vi "Balance_Sweep_Client.vi"(3 "Mode":bool, 4 "Measurement Time (ms)":i32, 5 "Stop Angle":dbl) -> (1 "Data Out":string)   [LabVIEW 2022 SP3]
uses:
  OGI_Server/ATE_Balance_Data.ctl
  Globals/Trav_pos_global.vi
  <vilib>/Platform/TimedLoop/XDataNode/XDataNode.xnode
  <vilib>/Platform/TimedLoop/XDataNode/timing_clust.ctl
  <vilib>/Platform/TimedLoop/XDataNode/wakeup.ctl
  <vilib>/Platform/TimedLoop/XDataNode/nitl_modes.ctl
  OGI_Server/ATE_Fan_Data.ctl
  <userlib>/LV-Link3/PolySubVIs/DtCreateAoutChan.vi
  <userlib>/LV-Link3/PolySubVIs/DtOLWriteSingle.vi
panel:
  out "Measurement Time":i32
  out "Initial":i64
  out "Target Angle":dbl
  out "Sampling Frequency":dbl
  out "DT Error":errorcluster
  out "Task out":i32
  out "Fan Data Ref":refnum<k21>
  out "Live Angle":dbl
  out "Balance Data Ref":refnum<k21>
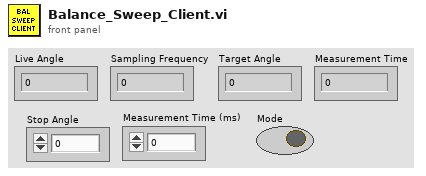
[diagram p1: front panel]
types:
  T1 = enum32{"Bad", "Idle", "Run top level", "Running"}
  T2 = typedef "XDNodeRunTimeDep.lvlib/timing_clust.ctl" = cluster{"Expected End [f-1]":u64, "Actual End [f-1]":u64, "Finished Late? [f-1]":bool, "Expected End [i-1]":u64, "Actual End [i-1]":u64, "Finished Late? [i-1]":bool, "Expected Start [i]":u64, "Actual Start [i]":u64, "Expected Start [f]":u64, "Actual Start [f]":u64, "Source Name":string, "Structure Name":string, "Period":i64, "Deadline":i64, "Offset":i64, "Start":i64, "Priority":i32, "Timeout":i32, "Mode":T3, "Wakeup Reason":T4, "Error":errorcluster, "Source Type":string, "Secondary Source Type":string, "Global End Time":u64, "Global Start Time":u64, "Frame Duration":u64, "Iteration Duration":u64, "Assigned CPU":i32, "I/O Scan Engine Mode":u32}
  T3 = typedef "XDNodeRunTimeDep.lvlib/nitl_modes.ctl" = enum32{"No Change", "Process missed periods, maintain original phase", "Discard missed periods, maintain original phase", "Process missed periods, ignore original phase", "Discard missed periods, ignore original phase"}
  T4 = typedef "XDNodeRunTimeDep.lvlib/wakeup.ctl" = enum32{"Normal", "Aborted", "Asynchronous wakeup", "Timing source error", "Timed loop error", "Timeout"}
  T5 = enum16{"big-endian, network order", "native, host order", "little-endian"}
  T6 = typedef "ATE_Fan_Data.ctl" = cluster{"Fan Speed (RPM)":dbl, "Wind Speed (m/s)":dbl, "SMAD Data":string}
  T7 = typedef "ATE_Balance_Data.ctl" = cluster{"%Lift":dbl, "Lift":dbl, "%Pitch":dbl, "Pitch":dbl, "%Drag":dbl, "Drag":dbl, "%Side":dbl, "Side":dbl, "%Yaw":dbl, "Yaw":dbl, "%Roll":dbl, "Roll":dbl}
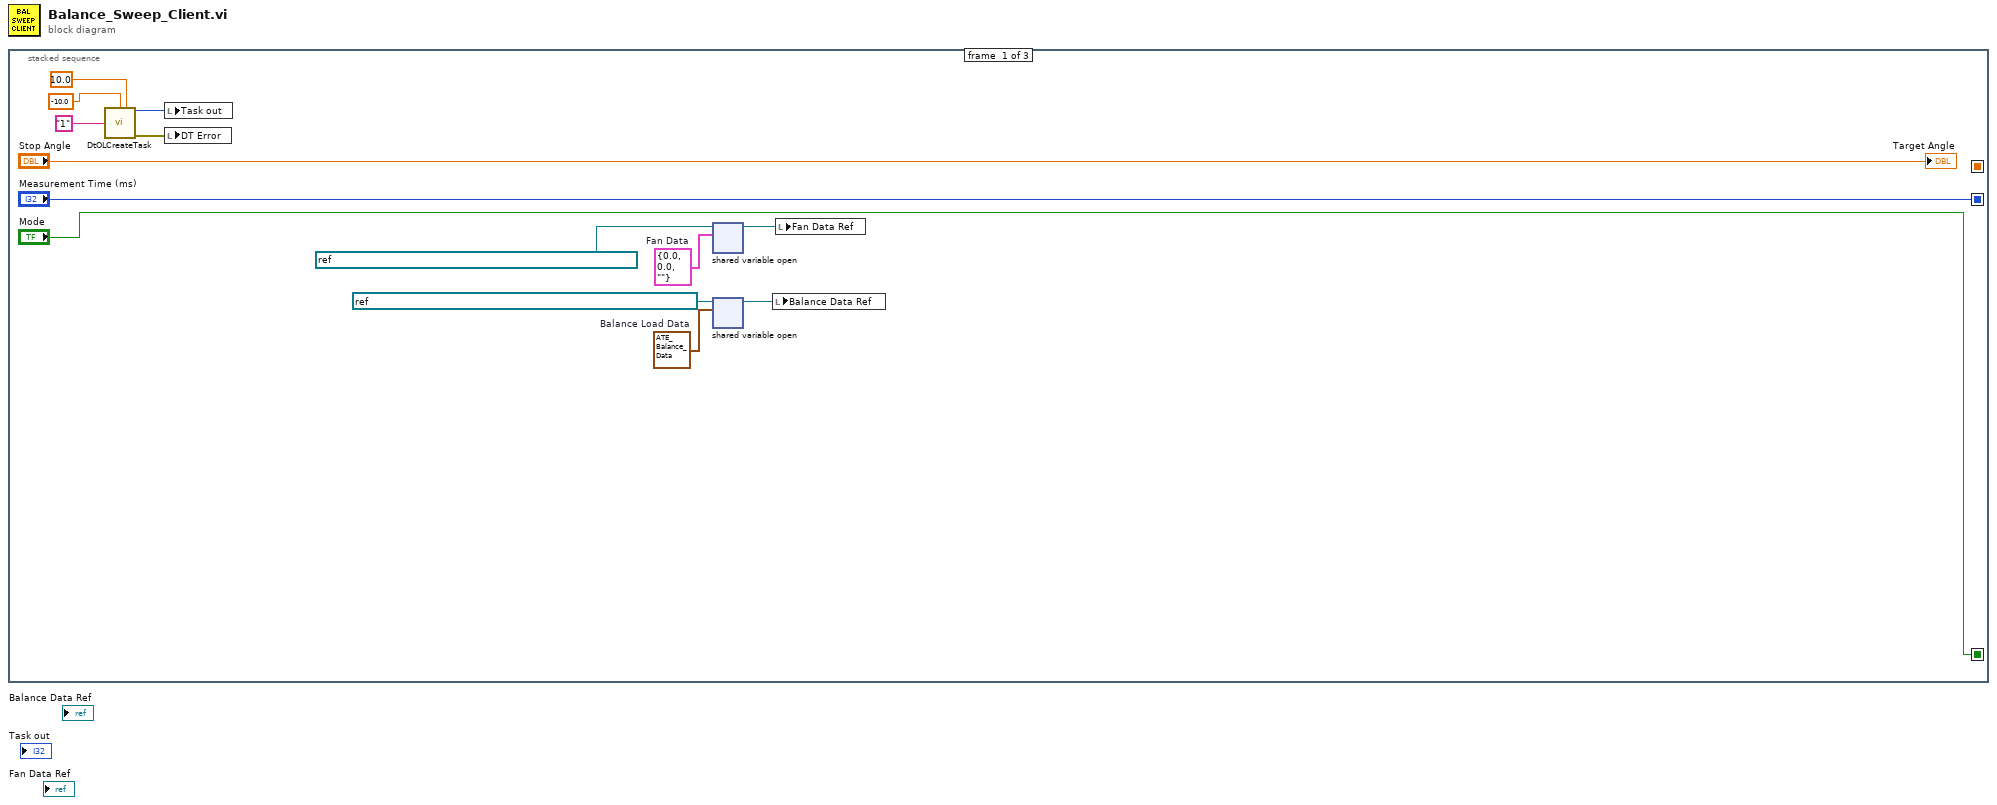
[diagram p0: block diagram]
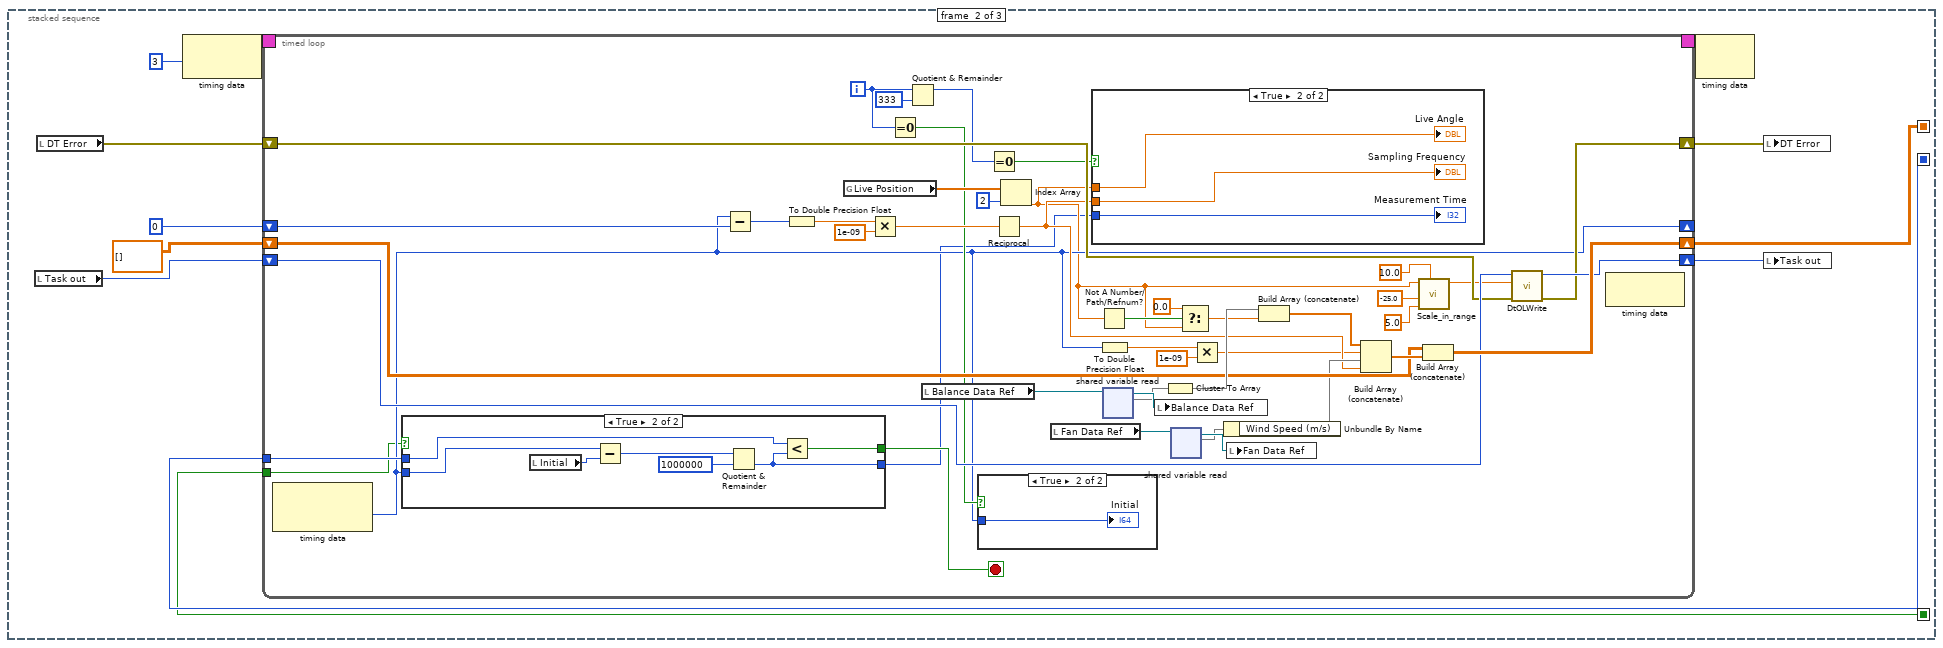
[diagram p2: hidden frame]
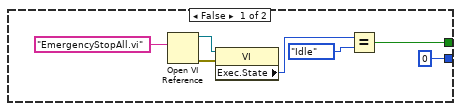
[diagram p5: hidden frame]
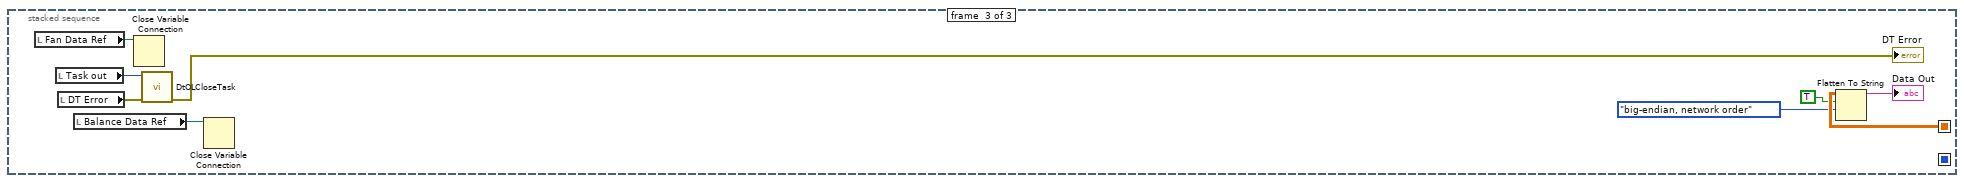
[diagram p6: hidden frame]
diagram:
  n1 = stacked-sequence {
    seq-local: [_ w23 _] -> [_ _ w104]
    seq-local: ["Measurement Time (ms)" _ _] -> [_ w16 _]
    seq-local: ["Mode" _ _] -> [_ w15 _]
    frame #0 {
      w10 = T6 {"Fan Speed (RPM)"=0.0, "Wind Speed (m/s)"=0.0, "SMAD Data"=""}  # Fan Data
      w13 = T7 {"%Lift"=0.0, "Lift"=0.0, "%Pitch"=0.0, "Pitch"=0.0, "%Drag"=0.0, "Drag"=0.0, "%Side"=0.0, "Side"=0.0, "%Yaw"=0.0, "Yaw"=0.0, "%Roll"=0.0, "Roll"=0.0}  # Balance Load Data
      n2 = call-poly <userlib>:"DtOLCreateTask.vi"("Range Min"=-10.0, "Range Max"=10.0, "Channel"="1") -> ("Task out"=w8:i32, "error out"=w4:errorcluster)  [unwired: 10 in, 1 out]
      n3 = local write "Task out"(w8) -> ()
      n4 = local write "DT Error"(w4) -> ()
      n5 = shared-variable-open(refnum<k21> "ni.var.psp://192.168.8.2/ATE_Shared_Variables/Fan_Data" ("shared variable refnum in"), w10) -> (w9:refnum<k21>)  [unwired: 2 in, 1 out]
      n6 = shared-variable-open(refnum<k21> "ni.var.psp://192.168.8.2/ATE_Shared_Variables/Balance_Data" ("shared variable refnum in"), w13) -> (w12:refnum<k21>)  [unwired: 2 in, 1 out]
      n7 = local write "Balance Data Ref"(w12) -> ()
      n8 = local write "Fan Data Ref"(w9) -> ()
      "Target Angle" <- "Stop Angle"
    }
    frame #1 {
      n9 = local read "Task out"() -> (w21:i32)
      n10 = local read "DT Error"() -> (w18:errorcluster)
      n11 = node-c288(i64 3 ("Period")) -> (w26:T2)
      n12 = timed-loop {
        timing: w26 -> [_]
        timing-out: [_] -> w25
        shift-right: [w64] -> w23
        shift-left: dbl[][] [] -> [w63]
        shift-right: [w55] -> w20
        shift-left: w21 -> [w56]
        shift-right: [w54] -> w19
        shift-left: w18 -> [w53]
        shift-right: [w35] -> _
        shift-left: i64 0 ("Global Start Time") -> [w52]
        tunnel: w16 -> [w37]
        tunnel: w15 -> [w28]
        i -> [w33]
        stop <- w57 stop-if-true
        n13 = node-c288() -> (w35:i64)  [unwired: 1 in, 1 out]
        n14 = case shown="True" w28 {
          tunnel: [w78 w84] -> w57
          tunnel: w37 -> [_ w85]
          tunnel: w35 -> [_ w89]
          tunnel: [i64 0 w83] -> w27
          frame False {
            n15 = Open VI Reference(vi path="EmergencyStopAll.vi") -> (vi reference=w81:refnum<vi>, error out=w80:errorcluster)  [unwired: 5 in]
            n16 = property class="VI"(reference=w81, error in=w80) -> ("Exec.State"=w77:T1)  [unwired: 2 out]
            n17 = Equal?(x=w77, y=T1."Idle") -> (x = y?=w78:bool)
          }
          frame True {
            n18 = local read "Initial"() -> (w88:i64)
            n19 = Subtract(x=w89, y=w88) -> (x-y=w87:i64)
            n20 = Quotient & Remainder(x=w87, y=i64 1000000) -> (floor(x/y)=w83:i64)  [unwired: 1 out]
            n21 = Less?(x=w85, y=w83) -> (x < y?=w84:bool)
          }
        }
        n22 = Subtract(x=w35, y=w52) -> (x-y=w51:i64)
        n23 = To Double Precision Float(number=w51) -> (double precision float=w49:dbl)
        n24 = global read "Trav_pos_global.vi" "Live Position"() -> (w69:sgl[])
        n25 = Multiply(x=w49, y=1e-09) -> (x*y=w44:dbl)
        n26 = Equal To 0?(x=w33) -> (x = 0?=w36:bool)
        n27 = Quotient & Remainder(x=w33, y=333) -> (x-y*floor(x/y)=w30:i32)  [unwired: 1 out]
        n28 = local read "Balance Data Ref"() -> (w71:refnum<k21>)
        n29 = case shown="True" w36 {
          tunnel: w35 -> [_ w75]
          frame False {
          }
          frame True {
            "Initial" <- w75
          }
        }
        n30 = Equal To 0?(x=w30) -> (x = 0?=w29:bool)
        n31 = Reciprocal(x=w44) -> (1/x=w48:dbl)
        n32 = Index Array(array=w69, index=2) -> (element=w31:sgl)
        n33 = local read "Fan Data Ref"() -> (w61:refnum<k21>)
        n34 = case shown="True" w29 {
          tunnel: w48 -> [_ w74]
          tunnel: w31 -> [_ w73]
          tunnel: w27 -> [_ w72]
          frame False {
          }
          frame True {
            "Sampling Frequency" <- w74
            "Live Angle" <- w73
            "Measurement Time" <- w72
          }
        }
        n35 = Not A Number/Path/Refnum?(number/path/refnum=w31) -> (NaN/Path/Refnum?=w41:bool)
        n36 = To Double Precision Float(number=w35) -> (double precision float=w47:dbl)
        n37 = shared-variable-read(w71) -> (w70:refnum<k21>, w67)  [unwired: 2 in, 2 out]
        n38 = local write "Balance Data Ref"(w70) -> ()
        n39 = Cluster To Array(cluster=w67) -> (array=w66:void[])
        n40 = shared-variable-read(w61) -> (w60:refnum<k21>, w59)  [unwired: 2 in, 2 out]
        n41 = Select(t=0.0, s=w41, f=w31) -> (s? t:f=w39:dbl)
        n42 = Multiply(x=w47, y=1e-09) -> (x*y=w45:dbl)
        n43 = Unbundle By Name(w59) -> ("Wind Speed (m/s)"=w58)
        n44 = local write "Fan Data Ref"(w60) -> ()
        n45 = Build Array (concatenate)(w66, w39) -> (w62:dbl[])
        n46 = Build Array (concatenate)(w62, w45, w58, w48) -> (w65:dbl[])
        n47 = call "Scale_in_range.vi"("Scale Factor"=10.0, "Maximum Range"=5.0, "Minimum Range"=-25.0, "x"=w31) -> ("Scaled x"=w40:dbl)  [unwired: 7 in]
        n48 = Build Array (concatenate)(w63, w65) -> (w64:dbl[][])
        n49 = call-poly <userlib>:"DtOLWrite.vi"("error in (no error)"=w53, "Data In"=w40, "Task in"=w56) -> ("error out"=w54:errorcluster, "Task out"=w55:i32)  [unwired: 7 in]
        n50 = node-c288() -> ()  [unwired: 1 in, 1 out]
      }
      n51 = node-c288(w25) -> ()  [unwired: 1 out]
      n52 = local write "DT Error"(w19) -> ()
      n53 = local write "Task out"(w20) -> ()
    }
    frame #2 {
      n54 = local read "Fan Data Ref"() -> (w100:refnum<k21>)
      n55 = local read "Task out"() -> (w99:i32)
      n56 = local read "DT Error"() -> (w98:errorcluster)
      n57 = local read "Balance Data Ref"() -> (w105:refnum<k21>)
      n58 = Close Variable Connection(11:w100) -> ()  [unwired: 1 in, 1 out]
      n59 = call <userlib>:"DtOLCloseTask.vi"("Error in"=w98, "Task in"=w99) -> ("Error Out"=→"DT Error":errorcluster)  [unwired: 9 in]
      n60 = Close Variable Connection(11:w105) -> ()  [unwired: 1 in, 1 out]
      n61 = Flatten To String(anything=w104, prepend array or string size? (T)=TRUE, byte order (0:big-endian, network order)=T5."big-endian, network order") -> (data string=→"Data Out":string)  [unwired: 1 in, 2 out]
    }
  }
